vi "Latch.vi"(11 "In":bool) -> (3 "Out":bool, 5 "button pressed":bool)   [LabVIEW 2016]
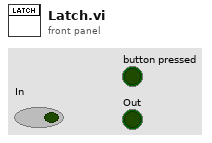
[diagram p1: front panel]
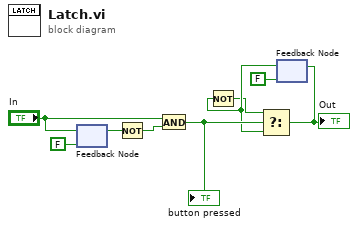
[diagram p0: block diagram]
diagram:
  n1 = feedback #1(FALSE) -> (w7:bool)
  n2 = feedback-in #1("In") -> ()
  n3 = Not(x=w7) -> (.not. x?=w8:bool)
  n4 = And(x="In", y=w8) -> (x .and. y?=w4:bool)
  "button pressed" <- w4
  n5 = feedback #2(FALSE) -> (w2:bool)
  n6 = Not(x=w2) -> (.not. x?=w1:bool)
  n7 = Select(t=w1, s=w4, f=w2) -> (s? t:f=w6:bool)
  "Out" <- w6
  n8 = feedback-in #2(w6) -> ()
